vi "Publish Status.vi"(8 "error in (no error)":errorcluster, 11 "Log Manager Module in":refnum<class "Log Manager Module.lvclass">) -> (0 "error out":errorcluster, 3 "Log Manager Module out":refnum<class "Log Manager Module.lvclass">)   [LabVIEW 2023, in "VolatusData.lvlib" / "Log Manager Module.lvclass"]
uses:
  Log Manager Module.lvclass
  Logger State.ctl
  Volatus/Module/Module.lvclass/Module.ctl
  Log Manager Module.lvclass/Log Manager Module.ctl
  Volatus/VolatusAPI/VolatusAPI.lvclass/VolatusAPI.ctl
  lv-vecto/Vecto/Group DBL/Group DBL.lvclass
  Volatus/VolatusAPI/Publish to Local Subs.vi
  VolatusData.lvlib
  Volatus/Module/Module.lvclass
  Volatus/VolatusAPI/VolatusAPI.lvclass
  C:/dev/volatus/mts-volatus-super/libs/lv-volatus/Volatus/Module/Module.lvclass
  C:/dev/volatus/mts-volatus-super/libs/lv-volatus/VolatusData/Log Manager Module/Log Manager Module.lvclass
  C:/dev/volatus/mts-volatus-super/libs/lv-vecto/Vecto/Group/Group.lvclass
  C:/dev/volatus/mts-volatus-super/libs/lv-vecto/Vecto/Group DBL/Group DBL.lvclass
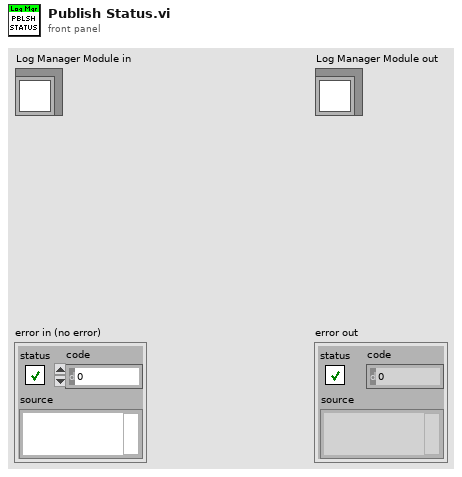
[diagram p1: front panel]
types:
  T1 = typedef "VolatusData.lvlib/Logger State.ctl" = enum16{"Unknown", "Idle", "Preparing", "Ready", "Logging", "Stopping"}
  T2 = typedef "VolatusData.lvlib/Logging State.ctl" = enum16{"Idle", "Starting", "Logging", "Stopping"}
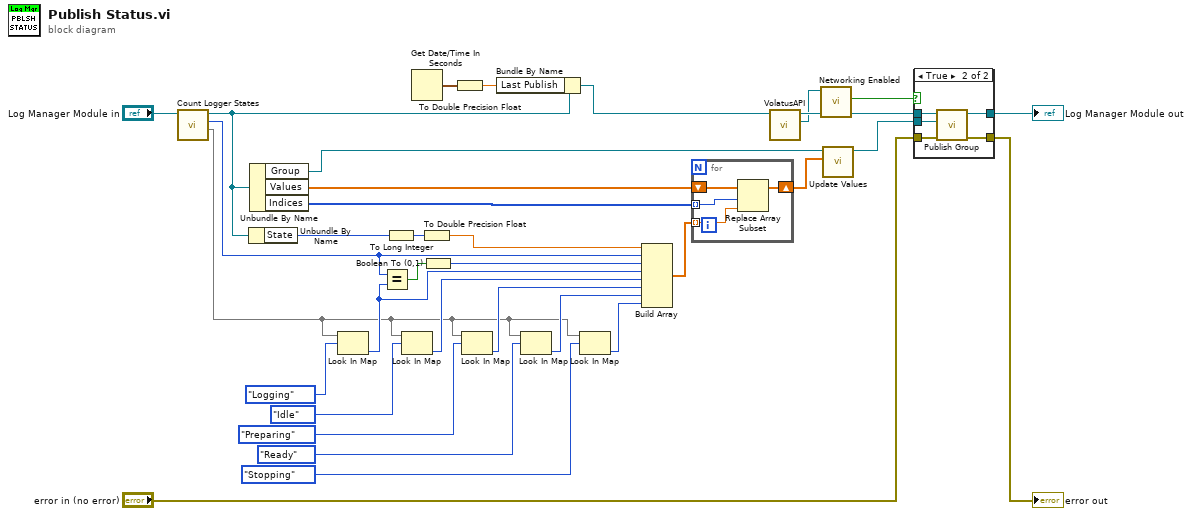
[diagram p0: block diagram]
diagram:
  n1 = call "Count Logger States.vi"("Log Manager Module in"="Log Manager Module in") -> ("Logger State Counts"=w10:map{T1, i32}, "Logger Count"=w9:i32, "Log Manager Module out"=w17:refnum<class "Log Manager Module.lvclass">)  [unwired: 7 in, 1 out]
  n2 = Unbundle By Name(w17) -> ("State"=w25:T2)
  n3 = Unbundle By Name(w17) -> ("Group"=w13:refnum<class "Group DBL.lvclass">, "Values"=w14:dbl[], "Indices"=w15:i32[])
  n4 = Look In Map(map=w10, key=Logger_State."Logging") -> (value=w22:i32)  [unwired: 1 in, 1 out]
  n5 = Equal?(x=w9, y=w22) -> (x = y?=w23:bool)
  n6 = To Long Integer(number=w25) -> (32bit integer=w26:i32)
  n7 = Look In Map(map=w10, key=Logger_State."Idle") -> (value=w21:i32)  [unwired: 1 in, 1 out]
  n8 = Get Date/Time In Seconds() -> (seconds since 1Jan1904=w2:timestamp)
  n9 = To Double Precision Float(number=w26) -> (double precision float=w24:dbl)
  n10 = Boolean To (0,1)(Boolean=w23) -> (0, 1=w4:i16)
  n11 = To Double Precision Float(number=w2) -> (double precision float=w1:dbl)
  n12 = Look In Map(map=w10, key=Logger_State."Preparing") -> (value=w20:i32)  [unwired: 1 in, 1 out]
  n13 = Bundle By Name(cluster=w17, "Last Publish"=w1) -> (w3:refnum<class "Log Manager Module.lvclass">)
  n14 = Look In Map(map=w10, key=Logger_State."Ready") -> (value=w19:i32)  [unwired: 1 in, 1 out]
  n15 = Look In Map(map=w10, key=Logger_State."Stopping") -> (value=w18:i32)  [unwired: 1 in, 1 out]
  n16 = Build Array(w24, w9, w4, w22, w21, w20, w19, w18) -> (w16:dbl[])
  n17 = for {
    tunnel: w16 -> [w36] mode=indexing
    tunnel: w15 -> [w37] mode=indexing
    shift-right: [w35] -> w12
    shift-left: w14 -> [w38]
    n18 = Replace Array Subset(array=w38, new element=w36, index=w37) -> (w35:dbl[])
  }
  n19 = call "VolatusAPI.vi"("Module in"=w3) -> ("VolatusAPI"=w6:refnum<class "VolatusAPI.lvclass">, "Module out"=w7:refnum<class "Log Manager Module.lvclass">)  [unwired: 9 in]
  n20 = call "Networking Enabled.vi"("VolatusAPI in"=w6) -> ("Networking Enabled"=w5:bool)  [unwired: 9 in, 1 out]
  n21 = call "Update Values.vi"("Values"=w12, "Group in"=w13) -> ("Group out"=w11:refnum<class "Group DBL.lvclass">)  [unwired: 8 in, 1 out]
  n22 = case shown="True" w5 {
    tunnel: [w40 w45] -> w29
    tunnel: "error in (no error)" -> [w39 w44]
    tunnel: [w39 w43] -> w27
    tunnel: w11 -> [_ w42]
    tunnel: w7 -> [w40 w41]
    frame False {
    }
    frame True {
      n23 = call "Publish Group.vi"("error in (no error)"=w44, "Group"=w42, "Module in"=w41) -> ("error out"=w43:errorcluster, "Module out"=w45:refnum<class "Log Manager Module.lvclass">)  [unwired: 7 in]
    }
  }
  "error out" <- w27
  "Log Manager Module out" <- w29
